vi "GetCmdParameters.vi"(3 "Contents":string) -> (1 "variables":string[](array[string]))   [LabVIEW 2012]
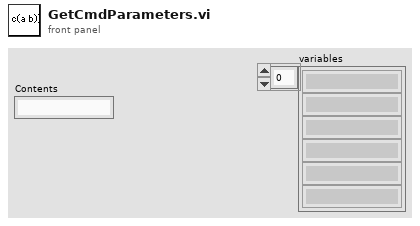
[diagram p1: front panel]
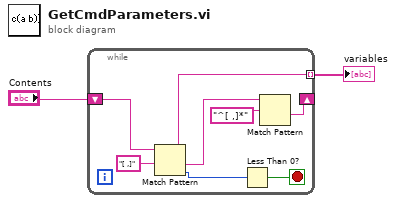
[diagram p0: block diagram]
diagram:
  n1 = while {
    tunnel: [w6] -> w1 mode=indexing
    shift-right: [w3] -> _
    shift-left: "Contents" -> [w10]
    stop <- w7 stop-if-true
    n2 = Match Pattern(string=w10, regular expression="[ ,]") -> (before substring=w6:string, after substring=w4:string, offset past match=w8:i32)  [unwired: 1 in, 1 out]
    n3 = Less Than 0?(x=w8) -> (x < 0?=w7:bool)
    n4 = Match Pattern(string=w4, regular expression="^[ ,]*") -> (after substring=w3:string)  [unwired: 1 in, 3 out]
  }
  "variables" <- w1
